vi "Get Manager.vi"(11 "Entity in":refnum<class "Entity.lvclass">) -> (2 "Entity Manager":refnum<class "Entity Manager.lvclass">)   [LabVIEW 2020, in "Conditum.lvlib" / "Entity.lvclass"]
uses:
  Entity.lvclass
  Entity.lvclass/Entity.ctl
  Entity Manager/Entity Manager.lvclass
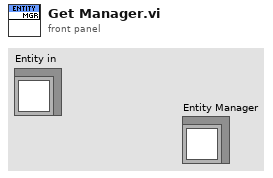
[diagram p1: front panel]
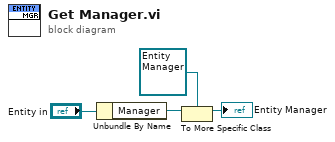
[diagram p0: block diagram]
diagram:
  n1 = Unbundle By Name("Entity in") -> ("Manager"=w3:refnum<class>)
  n2 = To More Specific Class(target class=refnum<class "Entity Manager.lvclass"> refnum ("Conditum:Entity Manager"), reference=w3) -> (specific class reference=→"Entity Manager":refnum<class "Entity Manager.lvclass">)  [unwired: 1 in, 1 out]
